vi "TDMStoASCII.vi"(8 "error in (no error)":errorcluster, 10 "Ascii file to write":path, 11 "TDMS File":path) -> (0 "error out":errorcluster)   [LabVIEW 2010, in "TDMS to ASCII Convert.lvlib"]
uses:
  TDMS to ASCII Convert.lvlib
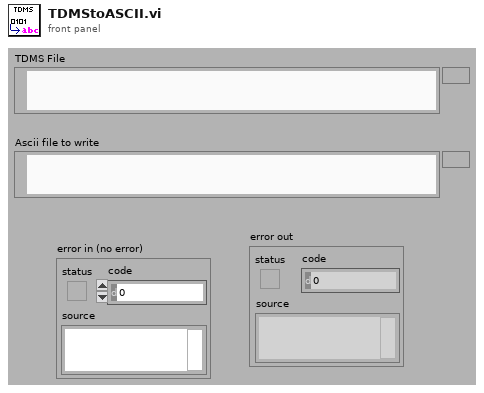
[diagram p1: front panel]
types:
  T1 = enum16{"open", "replace", "create", "open or create", "replace or create", "replace or create with confirmation"}
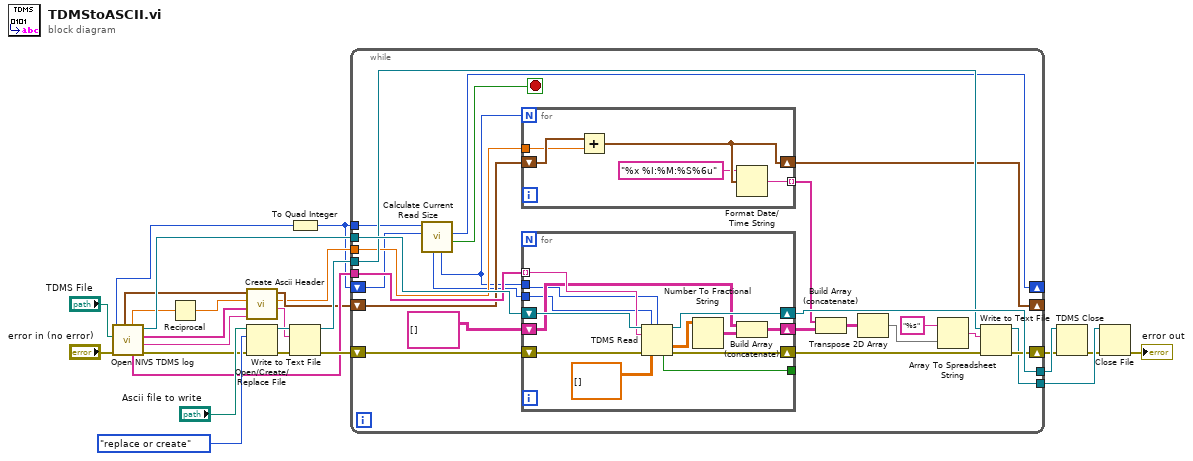
[diagram p0: block diagram]
diagram:
  n1 = call "Open NIVS TDMS log.vi"("error in (no error)"="error in (no error)", "TDMS File"="TDMS File") -> ("error out"=w18:errorcluster, "Log Name"=w9:string, "Sys Channel Names"=w8:string[], "tdms file out"=w24:refnum<k34>, "group names"=w6:string[], "Logging Rate"=w12:dbl, "Date Created"=w11:timestamp, "Datapoints"=w3:u32)  [unwired: 2 in]
  n2 = Reciprocal(x=w12) -> (1/x=w10:dbl)
  n3 = call "Create Ascii Header.vi"("Log Name"=w9, "Sys Channel Names"=w8, "Step Size"=w10, "Date Created"=w11) -> ("Header Spreadsheet String"=w7:string, "Step Size dup"=w4:dbl, "Date Created dup"=w5:timestamp)  [unwired: 5 in]
  n4 = Open/Create/Replace File(file path (use dialog)="Ascii file to write", error in=w18, operation (0:open)=T1."replace or create") -> (refnum out=w22:refnum<file>, error out=w19:errorcluster)  [unwired: 3 in, 1 out]
  n5 = To Quad Integer(1:w3) -> (0:w1:i64)
  n6 = Write to Text File(file (use dialog)=w22, text=w7, error in=w19) -> (refnum out=w13:refnum<file>, error out=w17:errorcluster)  [unwired: 1 in, 1 out]
  n7 = while {
    tunnel: [w50] -> w25
    tunnel: w24 -> [w49]
    shift-right: [w46] -> w15
    shift-left: w17 -> [w48]
    tunnel: [w45] -> w16
    tunnel: w13 -> [w44]
    tunnel: w6 -> [w43]
    tunnel: w4 -> [w40]
    shift-right: [w39] -> _
    shift-left: w5 -> [w41]
    shift-right: [w31] -> _
    shift-left: w1 -> [w32]
    tunnel: w1 -> [w30]
    stop <- w28 stop-if-true
    n8 = call "Calculate Current Read Size.vi"("Size Remaining in"=w32, "Total Size"=w30) -> ("Stop"=w28:bool, "Size Remaining out"=w31:i64, "Current Read Size"=w27:i64, "Offset"=w29:i64)  [unwired: 6 in]
    n9 = for {
      N: w27 -> [_]
      shift-right: [w54] -> w39
      shift-left: w41 -> [w55]
      tunnel: [w53] -> w36 mode=indexing
      tunnel: w40 -> [w51]
      n10 = Add(x=w55, y=w51) -> (x+y=w54:timestamp)
      n11 = Format Date/Time String(time format string (%c)="%x %I:%M:%S%6u", seconds (now)=w54) -> (date/time string=w53:string)  [unwired: 1 in]
    }
    n12 = for {
      tunnel: [w65] -> _
      shift-right: [w63] -> w47
      shift-left: w48 -> [w64]
      shift-right: [w68] -> w50
      shift-left: w49 -> [w67]
      tunnel: w43 -> [w62] mode=indexing
      shift-right: [w58] -> w35
      shift-left: string[][] [] -> [w60]
      tunnel: w27 -> [w57]
      tunnel: w29 -> [w56]
      n13 = TDMS Read(0:w67, 1:w56, 2:w57, 5:w62, 11:w64, 12:dbl[][] []) -> (4:w68:refnum<k34>, 10:w61:dbl[][], 14:w65:bool, 15:w63:errorcluster)  [unwired: 1 in, 2 out]
      n14 = Number To Fractional String(number=w61) -> (F-format string=w59:string[][])  [unwired: 3 in]
      n15 = Build Array (concatenate)(w60, w59) -> (w58:string[][])
    }
    n16 = Build Array (concatenate)(w36, w35) -> (w34:string[][])
    n17 = Transpose 2D Array(2D array=w34) -> (transposed array=w37:string[][])
    n18 = Array To Spreadsheet String(array=w37, 3:"%s" ("format string")) -> (spreadsheet string=w33:string)  [unwired: 1 in]
    n19 = Write to Text File(file (use dialog)=w44, text=w33, error in=w47) -> (refnum out=w45:refnum<file>, error out=w46:errorcluster)  [unwired: 1 in, 1 out]
  }
  n20 = TDMS Close(8:w15, 11:w25) -> (0:w14:errorcluster)  [unwired: 1 out]
  n21 = Close File(refnum=w16, error in=w14) -> (error out=→"error out":errorcluster)  [unwired: 1 out]
